vi "Execute.vi"(8 "error in (no error)":errorcluster, 11 "Measure in":refnum<class "Measure.lvclass">) -> (0 "error out":errorcluster, 2 "Test Result":refnum<class "Test Result.lvclass">, 3 "Measure out":refnum<class "Measure.lvclass">)   [LabVIEW 2021, in "Sequence Engine.lvlib" / "Measure.lvclass"]
uses:
  Measure.lvclass
  Test Result/Test Result.lvclass
  Test Result/Result Data.ctl
  Test Result/Test Status.ctl
  Measure.lvclass/Measure.ctl
  67e4c05b-29d7-41dd-b8f8-d9e712f9aa10.vi
  Sequence Engine.lvlib
panel:
  out "Aborted?":bool
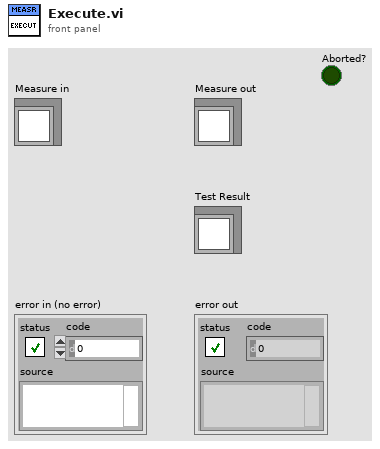
[diagram p1: front panel]
types:
  T1 = typedef "Sequence Engine.lvlib/Test Result.lvclass/Test Status.ctl" = enum16{"Pass", "Fail", "Aborted", "Skipped"}
  T2 = typedef "Sequence Engine.lvlib/Test Result.lvclass/Result Data.ctl" = cluster{"Test ID":u32, "Test Name":string, "Sub Test Name":string, "Test Status":T1, "Start Time":timestamp, "End Time":timestamp, "Duration (s)":dbl, "Expected Values":string, "Measured Values":string, "Remarks":string}
  T3 = typedef "Sequence Engine.lvlib/Broadcast Events--cluster.ctl" = cluster{"Module Did Init":refnum<user-event>, "Status Updated":refnum<user-event>, "Error Reported":refnum<user-event>, "Module Did Stop":refnum<user-event>, "Update Module Execution Status":refnum<user-event>, "New Test Result":refnum<user-event>, "Testing Started":refnum<user-event>, "Testing Completed":refnum<user-event>, "Retried Count":refnum<user-event>, "DUT Info":refnum<user-event>, "Stop Testing":refnum<user-event>}
  T4 = typedef "Sequence Engine.lvlib/Test Factory.lvclass/Test Config.ctl" = cluster{"Test ID":string, "Test Name":string, "Test Group":string, "Enabled?":bool, "Timeout (s)":u16, "Retry Count":u16, "Recipe Parameters":string, "Sequence Config":string}
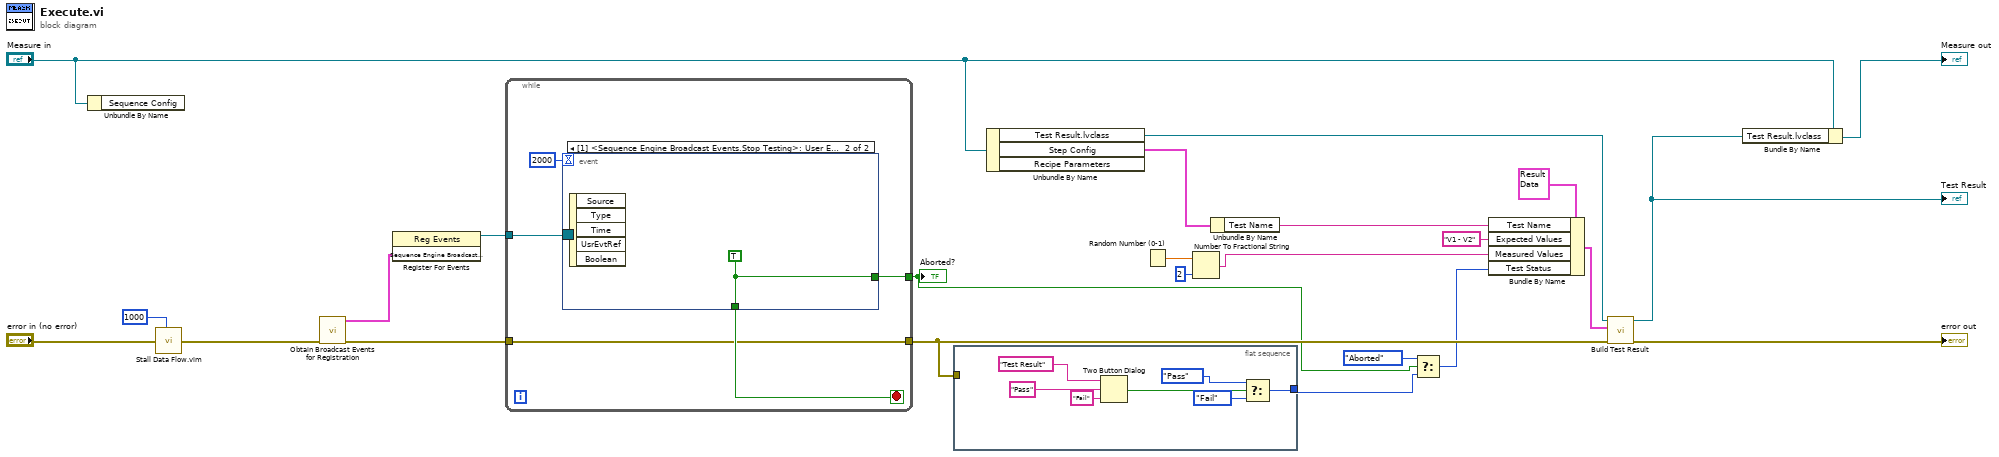
[diagram p0: block diagram]
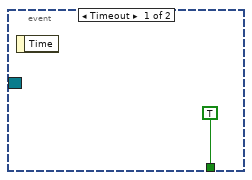
[diagram p2: hidden frame]
diagram:
  n1 = Unbundle By Name("Measure in") -> ()  [unwired: 1 out]
  n2 = call "Stall Data Flow.vim"("value in"="error in (no error)", "milliseconds to wait"=u32 1000) -> ("value out"=w22:errorcluster)  [unwired: 1 out]
  n3 = call "Obtain Broadcast Events for Registration.vi"("error in"=w22) -> ("error out"=w21:errorcluster, "Sequence Engine Broadcast Events"=w20:T3)  [unwired: 8 in, 1 out]
  n4 = register-events(w20) -> (reference out=w19:refnum<event-registration>)  [unwired: 2 in, 1 out]
  n5 = while {
    tunnel: w21 -> [w26]
    tunnel: w19 -> [w27]
    tunnel: [w26] -> w7
    tunnel: [w25] -> w3
    stop <- w28 stop-if-true
    n6 = event shown="[1] <Sequence Engine Broadcast Events.Stop Testing>: User Event" {
      selector: w27 -> [_ _]
      dyn-events: _ -> [_ _]
      timeout: 2000 -> [_ _]
      tunnel: [TRUE w31] -> w28
      tunnel: [_ w31] -> w25
      event Timeout {
        n7 = event-data() -> ()  [unwired: 1 in, 1 out]
      }
      event User Event {
        w31 = TRUE
        n8 = event-data() -> ()  [unwired: 1 in, 5 out]
      }
    }
  }
  "Aborted?" <- w3
  n9 = flat-sequence {
    tunnel: [w32] -> w5
    tunnel: w7 -> [_]
    frame #0 {
      n10 = Two Button Dialog(message="Test Result", 1:"Fail" ("F button name (\"Cancel\")"), 2:"Pass" ("T button name (\"OK\")")) -> (T button?=w34:bool)
      n11 = Select(t=Test_Status."Pass" ("Test Status"), s=w34, f=Test_Status."Fail") -> (s? t:f=w32:T1)
    }
  }
  n12 = Unbundle By Name("Measure in") -> ("Test Result.lvclass"=w16:refnum<class "Test Result.lvclass">, "Step Config"=w18:T4)  [unwired: 1 out]
  n13 = Random Number (0-1)() -> (number: 0 to 1=w8:dbl)
  n14 = Number To Fractional String(number=w8, precision (6)=i16 2) -> (F-format string=w9:string)  [unwired: 2 in]
  n15 = Unbundle By Name(w18) -> ("Test Name"=w17:string)
  n16 = Select(t=Test_Status."Aborted", s=w3, f=w5) -> (s? t:f=w4:T1)
  n17 = Bundle By Name(cluster=T2 {"Test ID"=0, "Test Name"="", "Sub Test Name"="", "Test Status"=enum."Pass", "Start Time"=timestamp(0 s since 1904-01-01), "End Time"=timestamp(0 s since 1904-01-01), "Duration (s)"=0.0, "Expected Values"="", "Measured Values"="", "Remarks"=""} ("Result Data"), "Test Name"=w17, "Expected Values"="V1 - V2", "Measured Values"=w9, "Test Status"=w4) -> (w14:T2)
  n18 = call "Build Test Result.vi"("error in (no error)"=w7, "Result Data"=w14, "Test Result in"=w16) -> ("error out"=→"error out":errorcluster, "Test Result out"=w13:refnum<class "Test Result.lvclass">)  [unwired: 7 in]
  "Test Result" <- w13
  n19 = Bundle By Name(cluster="Measure in", "Test Result.lvclass"=w13) -> (→"Measure out":refnum<class "Measure.lvclass">)
